vi "setEvaluation.vi"(8 "error in (no error)":errorcluster, 10 "evaluation":cluster{"F":dbl, "G":dbl, "H":dbl}, 11 "TreeNode in":refnum<class "TreeNode.lvclass">) -> (0 "error out":errorcluster, 3 "TreeNode out":refnum<class "TreeNode.lvclass">)   [LabVIEW 2009, in "TreeNode.lvclass"]
doc: "Sets the numerical evaluation of a node during a search."
uses:
  TreeNode.lvclass
  TreeNode.lvclass/TreeNode.ctl
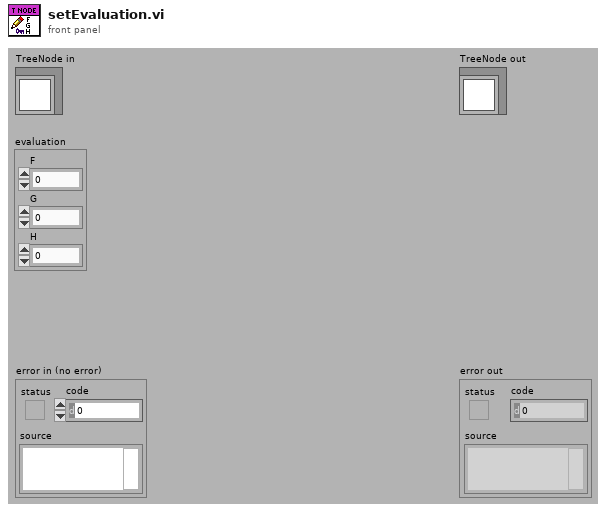
[diagram p1: front panel]
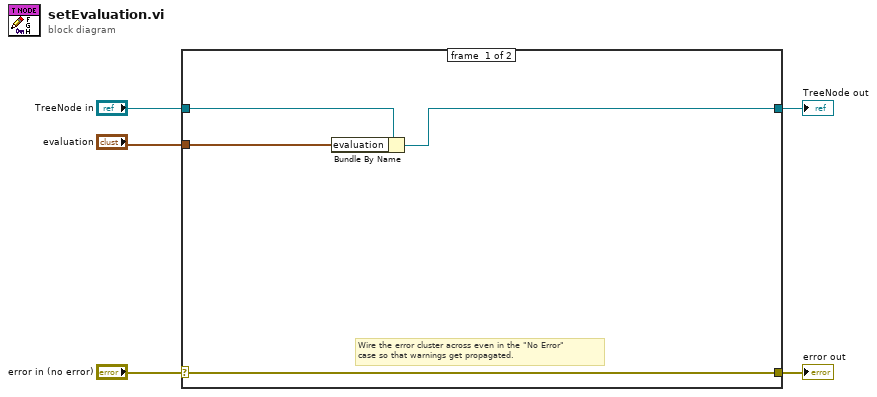
[diagram p0: block diagram]
diagram:
  n1 = case shown="No Error" "error in (no error)" {
    selector: "error in (no error)" -> [w9 w11]
    tunnel: [w9 w11] -> w4
    tunnel: [w7 w10] -> w2
    tunnel: "TreeNode in" -> [w8 w10]
    tunnel: "evaluation" -> [w6 _]
    frame #0 {
      # "Wire the error cluster across even in the \"No Error\"\ncase so that warnings get propagated."
      n2 = Bundle By Name(cluster=w8, "evaluation"=w6) -> (w7:refnum<class "TreeNode.lvclass">)
    }
    frame #1 {
    }
  }
  "error out" <- w4
  "TreeNode out" <- w2
